vi "test_fpga.vi"() -> ()   [LabVIEW 2016]
uses:
  FPGA Ref.ctl
  <vilib>/rvi/interface/nirviOpenFPGA/nirviOpenFPGA.xnode
  FPGA Bitfiles/SOAP.lvbitx
  <vilib>/FPGAPlugInAG/cRIO-9081/niLvFpga_Open_cRIO-9081.vi
  <vilib>/rvi/interface/nirviMethod/nirviMethod.xnode
  <vilib>/rvi/interface/nirviMethod/StockFPGA_InlinedMethodWaitForSingleIRQ.vi
  <vilib>/FPGAPlugInAG/cRIO-9081/niLvFpga_WaitOnIrq_cRIO-9081.vi
  <vilib>/FPGAPlugInAG/cRIO-9081/niLvFpga_AcknowledgeIrq_cRIO-9081.vi
  <vilib>/rvi/interface/nirviReadWriteControl/nirviReadWriteControl.xnode
  NiFpgaLv.dll
  <vilib>/Utility/error.llb/Error Cluster From Error Code.vi
  <vilib>/rvi/errors/niLvFpgaAdjustHostInterfaceError.vi
  <vilib>/Platform/TimedLoop/XDataNode/XDataNode.xnode
  <vilib>/Platform/TimedLoop/XDataNode/nitl_modes.ctl
  <vilib>/Platform/TimedLoop/XDataNode/XDNodeRunTimeDep.lvlib
  <vilib>/Platform/TimedLoop/XDataNode/wakeup.ctl
  <vilib>/Platform/TimedLoop/XDataNode/timing_clust.ctl
  <vilib>/rvi/interface/nirviCloseFPGA/nirviCloseFPGA.xnode
  <vilib>/FPGAPlugInAG/cRIO-9081/niLvFpga_Close_cRIO-9081.vi
  Controller/gController.lvclass
panel:
  in  "Stop Button":bool
  out "Sensor Status":u8
  out "double precision float":T1
  in  "error in":errorcluster
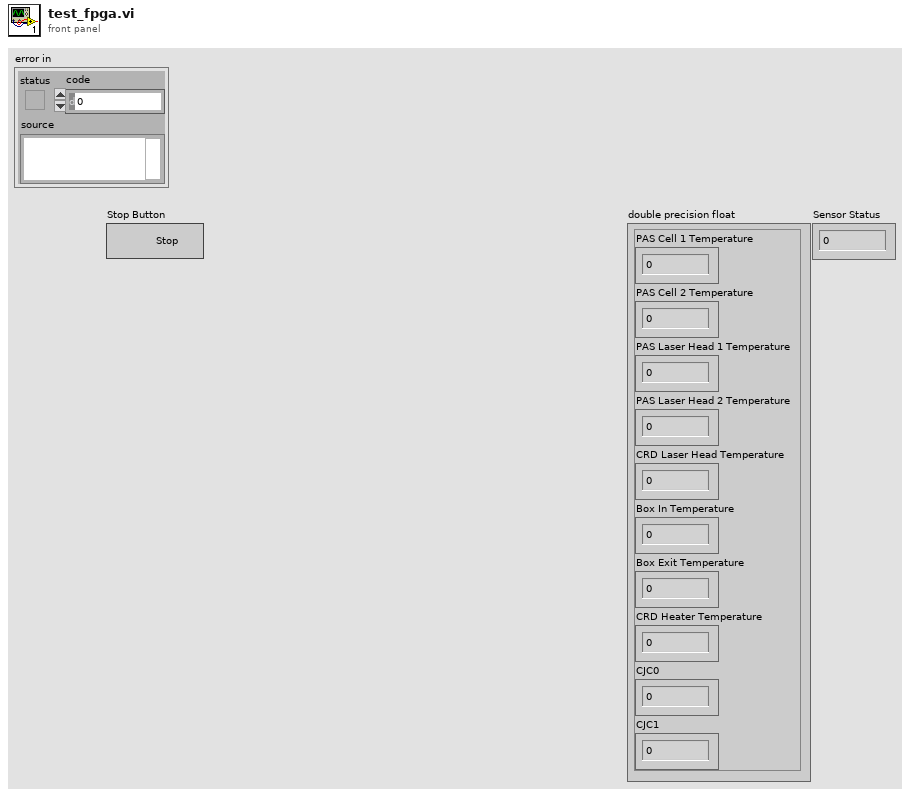
[diagram p1: front panel]
types:
  T1 = cluster{"PAS Cell 1 Temperature":dbl, "PAS Cell 2 Temperature":dbl, "PAS Laser Head 1 Temperature":dbl, "PAS Laser Head 2 Temperature":dbl, "CRD Laser Head Temperature":dbl, "Box In Temperature":dbl, "Box Exit Temperature":dbl, "CRD Heater Temperature":dbl, "CJC0":dbl, "CJC1":dbl}
  T2 = typedef "FPGA Ref.ctl" = refnum<k20>
  T3 = typedef "XDNodeRunTimeDep.lvlib/timing_clust.ctl" = cluster{"Expected End [f-1]":u64, "Actual End [f-1]":u64, "Finished Late? [f-1]":bool, "Expected End [i-1]":u64, "Actual End [i-1]":u64, "Finished Late? [i-1]":bool, "Expected Start [i]":u64, "Actual Start [i]":u64, "Expected Start [f]":u64, "Actual Start [f]":u64, "Source Name":string, "Structure Name":string, "Period":i64, "Deadline":i64, "Offset":i64, "Start":i64, "Priority":i32, "Timeout":i32, "Mode":T4, "Wakeup Reason":T5, "Error":errorcluster, "Source Type":string, "Secondary Source Type":string, "Global End Time":u64, "Global Start Time":u64, "Frame Duration":u64, "Iteration Duration":u64, "Assigned CPU":i32, "I/O Scan Engine Mode":u32}
  T4 = typedef "XDNodeRunTimeDep.lvlib/nitl_modes.ctl" = enum32{"No Change", "Process missed periods, maintain original phase", "Discard missed periods, maintain original phase", "Process missed periods, ignore original phase", "Discard missed periods, ignore original phase"}
  T5 = typedef "XDNodeRunTimeDep.lvlib/wakeup.ctl" = enum32{"Normal", "Aborted", "Asynchronous wakeup", "Timing source error", "Timed loop error", "Timeout"}
  T6 = cluster{"PAS Cell 1 Temperature":fxp<+/-,24,-2>, "PAS Cell 2 Temperature":fxp<+/-,24,-2>, "PAS Laser Head 1 Temperature":fxp<+/-,24,-2>, "PAS Laser Head 2 Temperature":fxp<+/-,24,-2>, "CRD Laser Head Temperature":fxp<+/-,24,-2>, "Box In Temperature":fxp<+/-,24,-2>, "Box Exit Temperature":fxp<+/-,24,-2>, "CRD Heater Temperature":fxp<+/-,24,-2>, "CJC0":fxp<+/-,24,-2>, "CJC1":fxp<+/-,24,-2>}
  T7 = cluster{"[0]":sgl, "[1]":sgl, "[2]":sgl, "[3]":sgl, "[4]":sgl, "[5]":sgl, "[6]":sgl, "[7]":sgl, "[8]":sgl, "[9]":sgl}
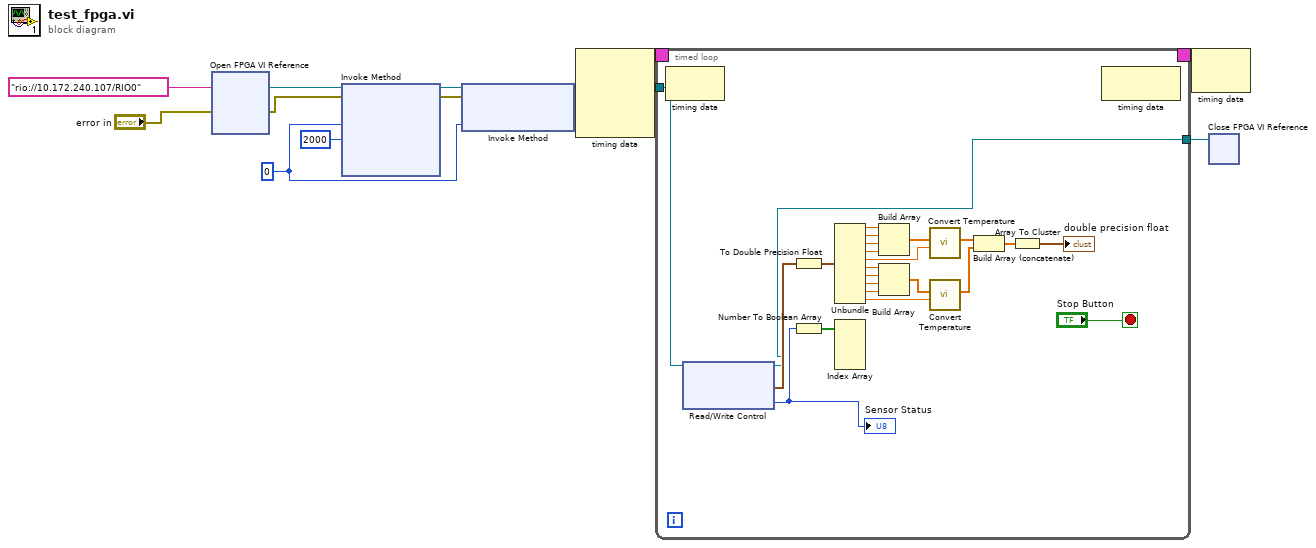
[diagram p0: block diagram]
diagram:
  w10 = 0 ("IRQ Number(s)")
  n1 = xnode "Open FPGA VI Reference"("error in"="error in", "resource name"=tag "rio://10.172.240.107/RIO0") -> ("FPGA VI Reference Out"=w11:T2, "error out"=w12:errorcluster)
  n2 = xnode "Invoke Method"("FPGA VI Reference In"=w11, "error in"=w12, "IRQ Number(s)"=w10, "Timeout (ms)"=2000) -> ("FPGA VI Reference Out"=w8:T2, "error out"=w9:errorcluster)  [unwired: 2 out]
  n3 = xnode "Invoke Method"("FPGA VI Reference In"=w8, "error in"=w9, "IRQ Number(s)"=w10) -> ("FPGA VI Reference Out"=w4:T2)  [unwired: 1 out]
  n4 = node-c288() -> (w3:T3)  [unwired: 4 in]
  n5 = timed-loop {
    tunnel: w4 -> [w16]
    timing: w3 -> [_]
    timing-out: [_] -> w2
    tunnel: [w15] -> w1
    stop <- "Stop Button" stop-if-true
    n6 = node-c288() -> ()  [unwired: 1 in, 1 out]
    n7 = xnode "Read/Write Control"("FPGA VI Reference In"=w16) -> ("FPGA VI Reference Out"=w15:T2, "Temperatures"=w18:T6, "Sensor Status"=w14:u8)  [unwired: 1 in, 1 out]
    "Sensor Status" <- w14
    n8 = To Double Precision Float(number=w18) -> (double precision float=w17:T1)
    n9 = Number To Boolean Array(number=w14) -> (Boolean array=w19:bool[])
    n10 = Unbundle(w17) -> ("PAS Cell 1 Temperature"=w31:dbl, "PAS Cell 2 Temperature"=w30:dbl, "PAS Laser Head 1 Temperature"=w29:dbl, "PAS Laser Head 2 Temperature"=w28:dbl, "CRD Laser Head Temperature"=w27:dbl, "Box In Temperature"=w25:dbl, "Box Exit Temperature"=w24:dbl, "CRD Heater Temperature"=w23:dbl, "CJC0"=w22:dbl, "CJC1"=w21:dbl)
    n11 = Index Array(array=w19) -> ()  [unwired: 4 in, 4 out]
    n12 = Build Array(w31, w30, w29, w28) -> (w26:dbl[])
    n13 = Build Array(w25, w24, w23, w22) -> (w20:dbl[])
    n14 = call "Convert Temperature.vi"("CJC"=w27, "TC Input"=w26) -> ("Temperature"=w34:sgl[])  [unwired: 9 in]
    n15 = call "Convert Temperature.vi"("CJC"=w21, "TC Input"=w20) -> ("Temperature"=w33:sgl[])  [unwired: 9 in]
    n16 = Build Array (concatenate)(w34, w33) -> (w32:sgl[])
    n17 = Array To Cluster(array=w32) -> (cluster=→"double precision float":T7)
    n18 = node-c288() -> ()  [unwired: 1 in, 1 out]
  }
  n19 = node-c288(w2) -> ()  [unwired: 1 out]
  n20 = xnode "Close FPGA VI Reference"("FPGA VI Reference In"=w1) -> ()  [unwired: 1 in, 1 out]
